vi "BIO_puts.vi"(7 "Timeout (10000ms)":u32=10000, 8 "error in (no error)":errorcluster, 10 "String to write":string, 11 "BIO in":refnum<class "BIO.lvclass">) -> (0 "error out":errorcluster, 3 "BIO out":refnum<class "BIO.lvclass">)   [LabVIEW 2013, in "SSL_Lib.lvlib" / "BIO.lvclass"]
uses:
  BIO.lvclass
  SSL-Lib/SSL-Lib.lvclass
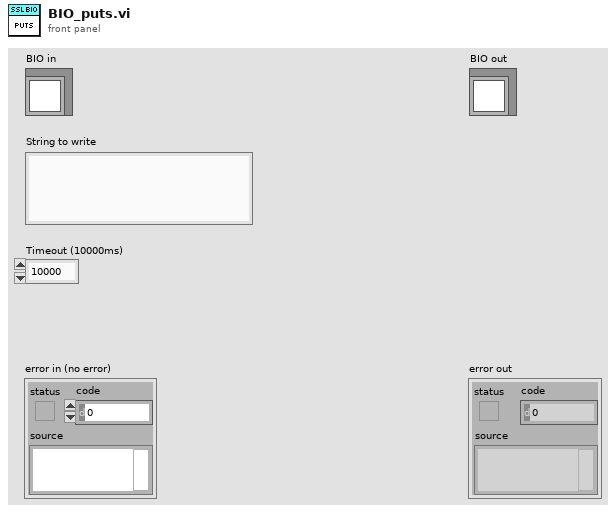
[diagram p1: front panel]
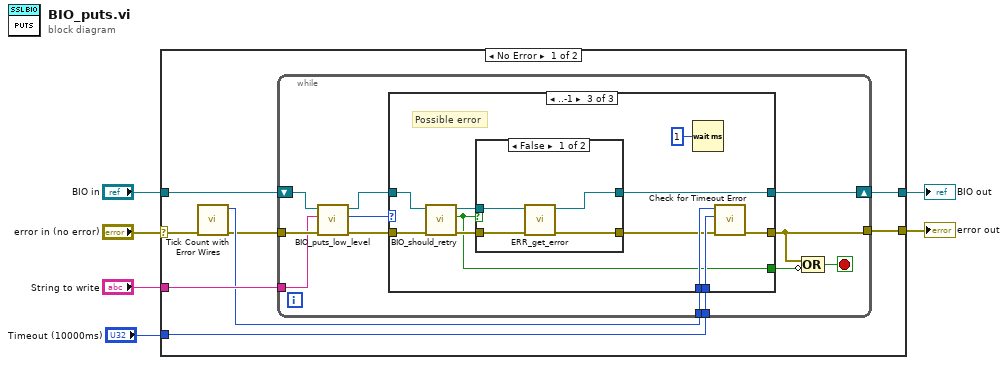
[diagram p0: block diagram]
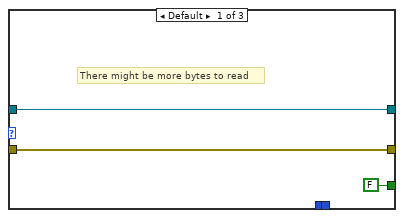
[diagram p2: hidden frame]
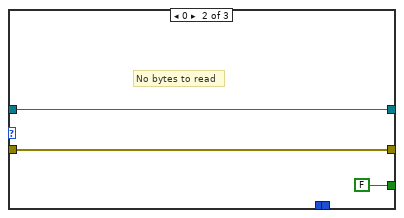
[diagram p3: hidden frame]
diagram:
  n1 = case shown="No Error" "error in (no error)" {
    selector: "error in (no error)" -> [w11 w51]
    tunnel: [w12 w51] -> w5
    tunnel: [w13 w50] -> w3
    tunnel: "BIO in" -> [w7 w50]
    tunnel: "String to write" -> [w14 _]
    tunnel: "Timeout (10000ms)" -> [w9 _]
    frame No Error {
      n2 = call "Tick Count with Error Wires.vi"("error in (no error)"=w11) -> ("error out"=w8:errorcluster, "millisecond timer value"=w10:u32)  [unwired: 9 in]
      n3 = while {
        tunnel: w14 -> [w15]
        shift-right: [w24] -> w13
        shift-left: w7 -> [w16]
        tunnel: w8 -> [w26]
        tunnel: [w22] -> w12
        tunnel: w10 -> [w20]
        tunnel: w9 -> [w19]
        stop <- w21 stop-if-true
        n4 = call "BIO_puts_low_level.vi"("error in (no error)"=w26, "String to write"=w15, "BIO in"=w16) -> ("error out"=w25:errorcluster, "return type"=w18:i32, "BIO out"=w17:refnum<class "BIO.lvclass">)  [unwired: 6 in]
        n5 = case shown="..-1" w18 {
          tunnel: w25 -> [w28 w32 w43]
          tunnel: [w28 w32 w36] -> w22
          tunnel: w17 -> [w29 w31 w42]
          tunnel: [w29 w31 w39] -> w24
          tunnel: [FALSE ("Should retry") FALSE w33] -> w23
          tunnel: w20 -> [_ _ w37]
          tunnel: w19 -> [_ _ w38]
          frame Default {
            # "There might be more bytes to read"
          }
          frame 0 {
            # "No bytes to read"
          }
          frame ..-1 {
            # "Possible error"
            n6 = call "BIO_should_retry.vi"("error in (no error)"=w43, "BIO in"=w42) -> ("error out"=w41:errorcluster, "Should retry"=w33:bool, "BIO out"=w40:refnum<class "BIO.lvclass">)  [unwired: 7 in]
            n7 = case shown="False" w33 {
              tunnel: w41 -> [w47 w48]
              tunnel: [w46 w48] -> w35
              tunnel: w40 -> [w45 w49]
              tunnel: [w44 w49] -> w39
              frame False {
                n8 = call "ERR_get_error.vi"("error in (no error)"=w47, "SSL-Lib in"=w45) -> ("error out"=w46:errorcluster, "SSL-Lib out"=w44:refnum<class "BIO.lvclass">)  [unwired: 8 in]
              }
              frame True {
              }
            }
            n9 = Wait (ms)(milliseconds to wait=u32 1) -> ()  [unwired: 1 out]
            n10 = call "Check for Timeout Error.vi"("error in (no error)"=w35, "Timeout (10000ms)"=w38, "t0"=w37) -> ("error out"=w36:errorcluster)  [unwired: 8 in]
          }
        }
        n11 = Compound Arithmetic op=OR(w22, invert w23) -> (w21:bool)
      }
    }
    frame Error {
    }
  }
  "error out" <- w5
  "BIO out" <- w3
